vi "CLD 13 Timer w flow sensitivity.vi"(8 "Fehler (Eingang)":T1, 10 "Flussrate":i8(slide) min=-2 max=2 step=1 scale=-2.0..2.0, 11 "Timer-Enum":T2) -> (0 "Fehler (Ausgang)":T1, 3 "Verstrichene Zeit":dbl)   [LabVIEW 2014]
doc: "CLD 13 - Dieser Timer setzt sich selbst zurück, wenn die eingehende Flussrate gleich null ist."
uses:
  CLD 13 timer Enum.ctl
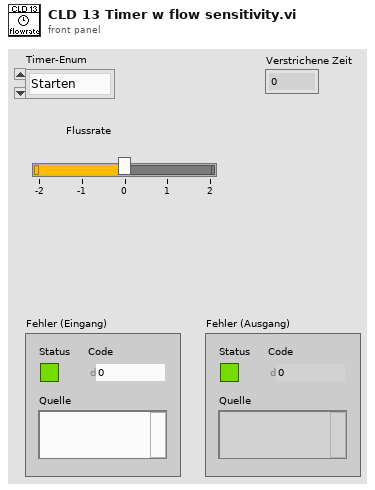
[diagram p1: front panel]
types:
  T1 = cluster{"Status":bool, "Code":i32, "Quelle":string}
  T2 = typedef "CLD 13 timer Enum.ctl" = enum16{"Starten", "Lesen"}
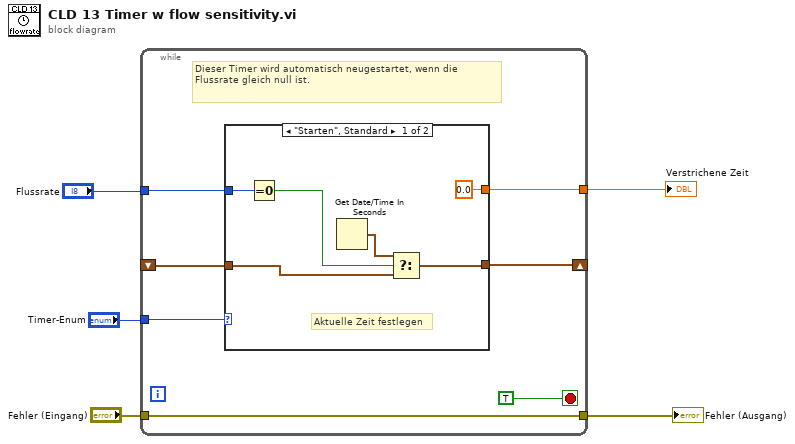
[diagram p0: block diagram]
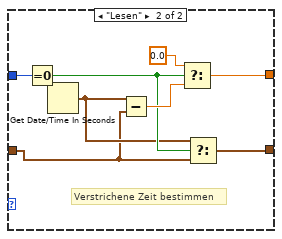
[diagram p2: hidden frame]
diagram:
  n1 = while {
    tunnel: "Timer-Enum" -> [w11]
    shift-right: [w10] -> _
    shift-left: _ -> [w9]
    tunnel: [w8] -> w4
    tunnel: "Flussrate" -> [w7]
    tunnel: [w6] -> w1
    tunnel: "Fehler (Eingang)" -> [w6]
    stop <- TRUE stop-if-true
    # "Dieser Timer wird automatisch neugestartet, wenn die Flussrate gleich null ist."
    n2 = case shown="\"Starten\", Standard" w11 {
      tunnel: [w14 w19] -> w10
      tunnel: w9 -> [w13 w20]
      tunnel: [0.0 w25] -> w8
      tunnel: w7 -> [w17 w23]
      frame "Starten", Default {
        # "Aktuelle Zeit festlegen"
        n3 = Equal To 0?(x=w17) -> (x = 0?=w16:bool)
        n4 = Get Date/Time In Seconds() -> (seconds since 1Jan1904=w15:timestamp)
        n5 = Select(t=w15, s=w16, f=w13) -> (s? t:f=w14:timestamp)
      }
      frame "Lesen" {
        # "Verstrichene Zeit bestimmen"
        n6 = Equal To 0?(x=w23) -> (x = 0?=w22:bool)
        n7 = Get Date/Time In Seconds() -> (seconds since 1Jan1904=w21:timestamp)
        n8 = Subtract(x=w21, y=w20) -> (x-y=w26:dbl)
        n9 = Select(t=0.0, s=w22, f=w26) -> (s? t:f=w25:dbl)
        n10 = Select(t=w21, s=w22, f=w20) -> (s? t:f=w19:timestamp)
      }
    }
  }
  "Verstrichene Zeit" <- w4
  "Fehler (Ausgang)" <- w1
